vi "apply channel changes.vi"(8 "error in":errorcluster, 9 "new":refnum<class "TBM channel.lvclass">, 10 "old":refnum<class "TBM channel.lvclass">, 11 "Scan Engine configuration":refnum<class "Scan Engine configuration.lvclass">) -> (0 "error out":errorcluster, 3 "Scan Engine configuration out":refnum<class "Scan Engine configuration.lvclass">)   [LabVIEW 2013, in "Scan Engine configuration.lvclass"]
uses:
  Scan Engine configuration.lvclass
  <vilib>/NI/Tag Bus Module Framework/channel/TBM channel.lvclass
  Scan Engine configuration.lvclass/Scan Engine configuration.ctl
  <vilib>/NI/Tag Bus/tag/tag descriptor.lvclass/tag descriptor.ctl
  <vilib>/NI/Tag Bus/tag/read tag name.vi
  <vilib>/NI/Tag Bus/tag/tag descriptor.lvclass
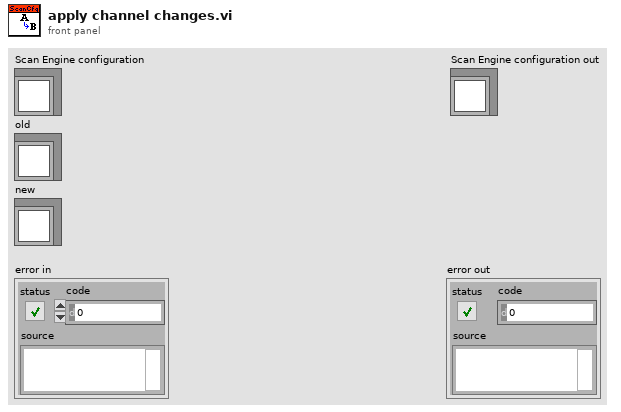
[diagram p1: front panel]
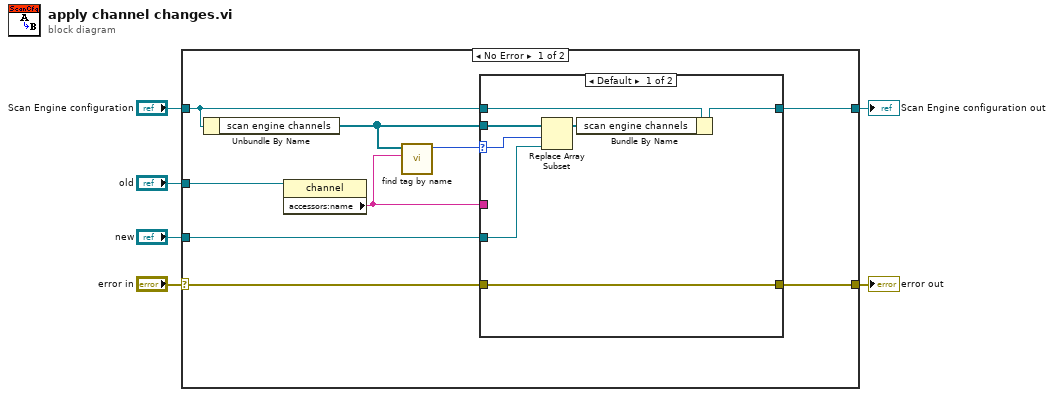
[diagram p0: block diagram]
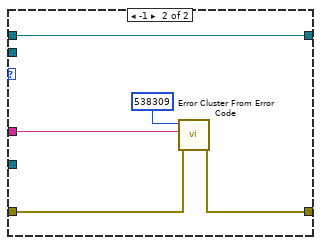
[diagram p2: hidden frame]
diagram:
  n1 = case shown="No Error" "error in" {
    selector: "error in" -> [w11 w29]
    tunnel: [w10 w29] -> w1
    tunnel: [w14 w28] -> w2
    tunnel: "Scan Engine configuration" -> [w15 w28]
    tunnel: "new" -> [w8 _]
    tunnel: "old" -> [w7 _]
    frame No Error {
      n2 = Unbundle By Name(w15) -> ("scan engine channels"=w13:refnum<class "TBM channel.lvclass">[])
      n3 = property class="channel"(reference=w7) -> ("accessors:name"=w12:string)  [unwired: 1 in, 2 out]
      n4 = call <vilib>:"find tag by name.vi"("name"=w12, "tags in"=w13) -> ("index"=w9:i32)  [unwired: 9 in]
      n5 = case shown="Default" w9 {
        selector: w9 -> [w20 _]
        tunnel: w15 -> [w22 w27]
        tunnel: [w19 w27] -> w14
        tunnel: w13 -> [w21 _]
        tunnel: w8 -> [w17 _]
        tunnel: w12 -> [_ w25]
        tunnel: w11 -> [w16 w24]
        tunnel: [w16 w23] -> w10
        frame Default {
          n6 = Replace Array Subset(array=w21, new element=w17, index=w20) -> (w18:refnum<class "TBM channel.lvclass">[])
          n7 = Bundle By Name(cluster=w22, "scan engine channels"=w18) -> (w19:refnum<class "Scan Engine configuration.lvclass">)
        }
        frame -1 {
          n8 = call <vilib>:"Error Cluster From Error Code.vi"("error in (no error)"=w24, "error message (\"\")"=w25, "error code (0)"=538309) -> ("error out"=w23:errorcluster)  [unwired: 6 in]
        }
      }
    }
    frame Error {
    }
  }
  "Scan Engine configuration out" <- w2
  "error out" <- w1
